vi "Sandbox HI Press.vi"() -> ()   [LabVIEW 2019]
uses:
  FPGA_API_class/FPGA API.lvclass
  FPGA/TypeDef/DO index.ctl
  <vilib>/Platform/TimedLoop/XDataNode/timing_clust.ctl
  <vilib>/Platform/TimedLoop/XDataNode/nitl_modes.ctl
  <vilib>/Platform/TimedLoop/XDataNode/wakeup.ctl
  Database_Postgress_class/Database_Postgress.lvclass
  D:/H4000/src/DatabaseInterface_class/DatabaseInterface.lvclass
  Database_Postgress_class/Connection Info.ctl
  Logger_class/Logger.lvclass
  ConfigJSON_class/ConfigJSON.lvclass
  D:/H4000/src/ConfigInterface_class/ConfigInterface.lvclass
  ConfigJSON_class/ConfigJSON.lvclass/ConfigJSON.ctl
  MessageAMC_class/MessageAMC.lvclass
  D:/H4000/src/MessageInterface_class/MessageInterface.lvclass
  Sig_AI_class/Sig_AI.lvclass
  D:/H4000/src/Proccess_class/Proccess.lvclass
  Sig_AI_class/Sig_AI.lvclass/Sig_AI.ctl
  Proccess_class/Proccess.lvclass/Proccess.ctl
  Logger_class/Logger.lvclass/Logger.ctl
  AnalogComparator_class/AnalogComparator.lvclass/AnalogComparator.ctl
  f5bc6a8b-969d-497a-8a5c-051cf4284504.vi
  ecb9b5e4-2695-48ff-9181-73dd1b10c553.vi
  af552bff-813f-42b3-9aac-38add1df6ad3.vi
  598a9a7a-3cbd-43cc-b63b-695f4522b225.vi
  Sig_AI_class/private/WriteToDb.vi
  Sig_AI_class/HandleRanges.vi
  Sig_AI_class/HandleAlarms.vi
  subvis/Scale_Raw_to_EU.vi
  AnalogComparator_class/GetStatus.vi
  AnalogComparator_class/GetTh.vi
  Logger_class/Enqueue Signal.vi
  Proccess_class/Read TagName.vi
  Proccess_class/Read Logger.vi
  AnalogComparator_class/SetValue.vi
  AnalogComparator_class/HandleDb.vi
  <vilib>/platform/TimedLoop/XDataNode/XDataNode.xnode
  <vilib>/Platform/TimedLoop/XDataNode/XDNodeRunTimeDep.lvlib
  Proccess_class/Proccess.lvclass
  DatabaseInterface_class/DatabaseInterface.lvclass
  <vilib>/ptbypt/NI_PtbyPt.lvlib
panel:
  in  "Time, ms":u32
  in  "Impulse open":bool
  out "x > y? 2":bool
  out "x > y?":bool
  out "Waveform Chart 4":dbl[][](graph)
  out "Waveform Chart 3":dbl(graph)
  out "Waveform Chart 2":dbl[][](graph)
  out "error out":errorcluster
  out "Iteration Duration":i64
  in  "Enable Stop Drive":bool
  in  "Enable Close Outlet":bool
  in  "Enable Close Inlet":bool
  out "SP RAW":dbl
  out "Waveform Chart":cluster{"SP":dbl, "Scaled":dbl}(graph)
  out "AI 6":dbl caption="Давление в образце\n[AI 6]"
  out "AI 5":dbl caption="Давление после насоса \nвысокого давления [AI 5]"
  out "AI 9":dbl caption="Давление  в  линии подачи \nвоздуха после БПВ [AI 9]"
  out "AI 8":dbl caption="Давление  в  линии подачи \nвоздуха в БПВ [AI 8]"
  out "AI4":dbl caption="ОС от клапана \n[AI 4]"
  out "DO 14":bool caption="Y29.10  \n33.6\nDO14"
  out "DO 17":bool caption="33.3\nY29.13\nDO17"
  out "DO 6":bool caption="33.8\nY29.2\nDO6"
  out "DO 9":bool caption="33.1\nY29.5\nDO9"
  out "19":bool caption="AIR"
  in  "SP 2":dbl
  in  "stop":bool
  in  "ALARM":bool
  in  "SP":dbl
  in  "GO DOWN":bool
  in  "GP UP":bool
  in  "AIR":bool
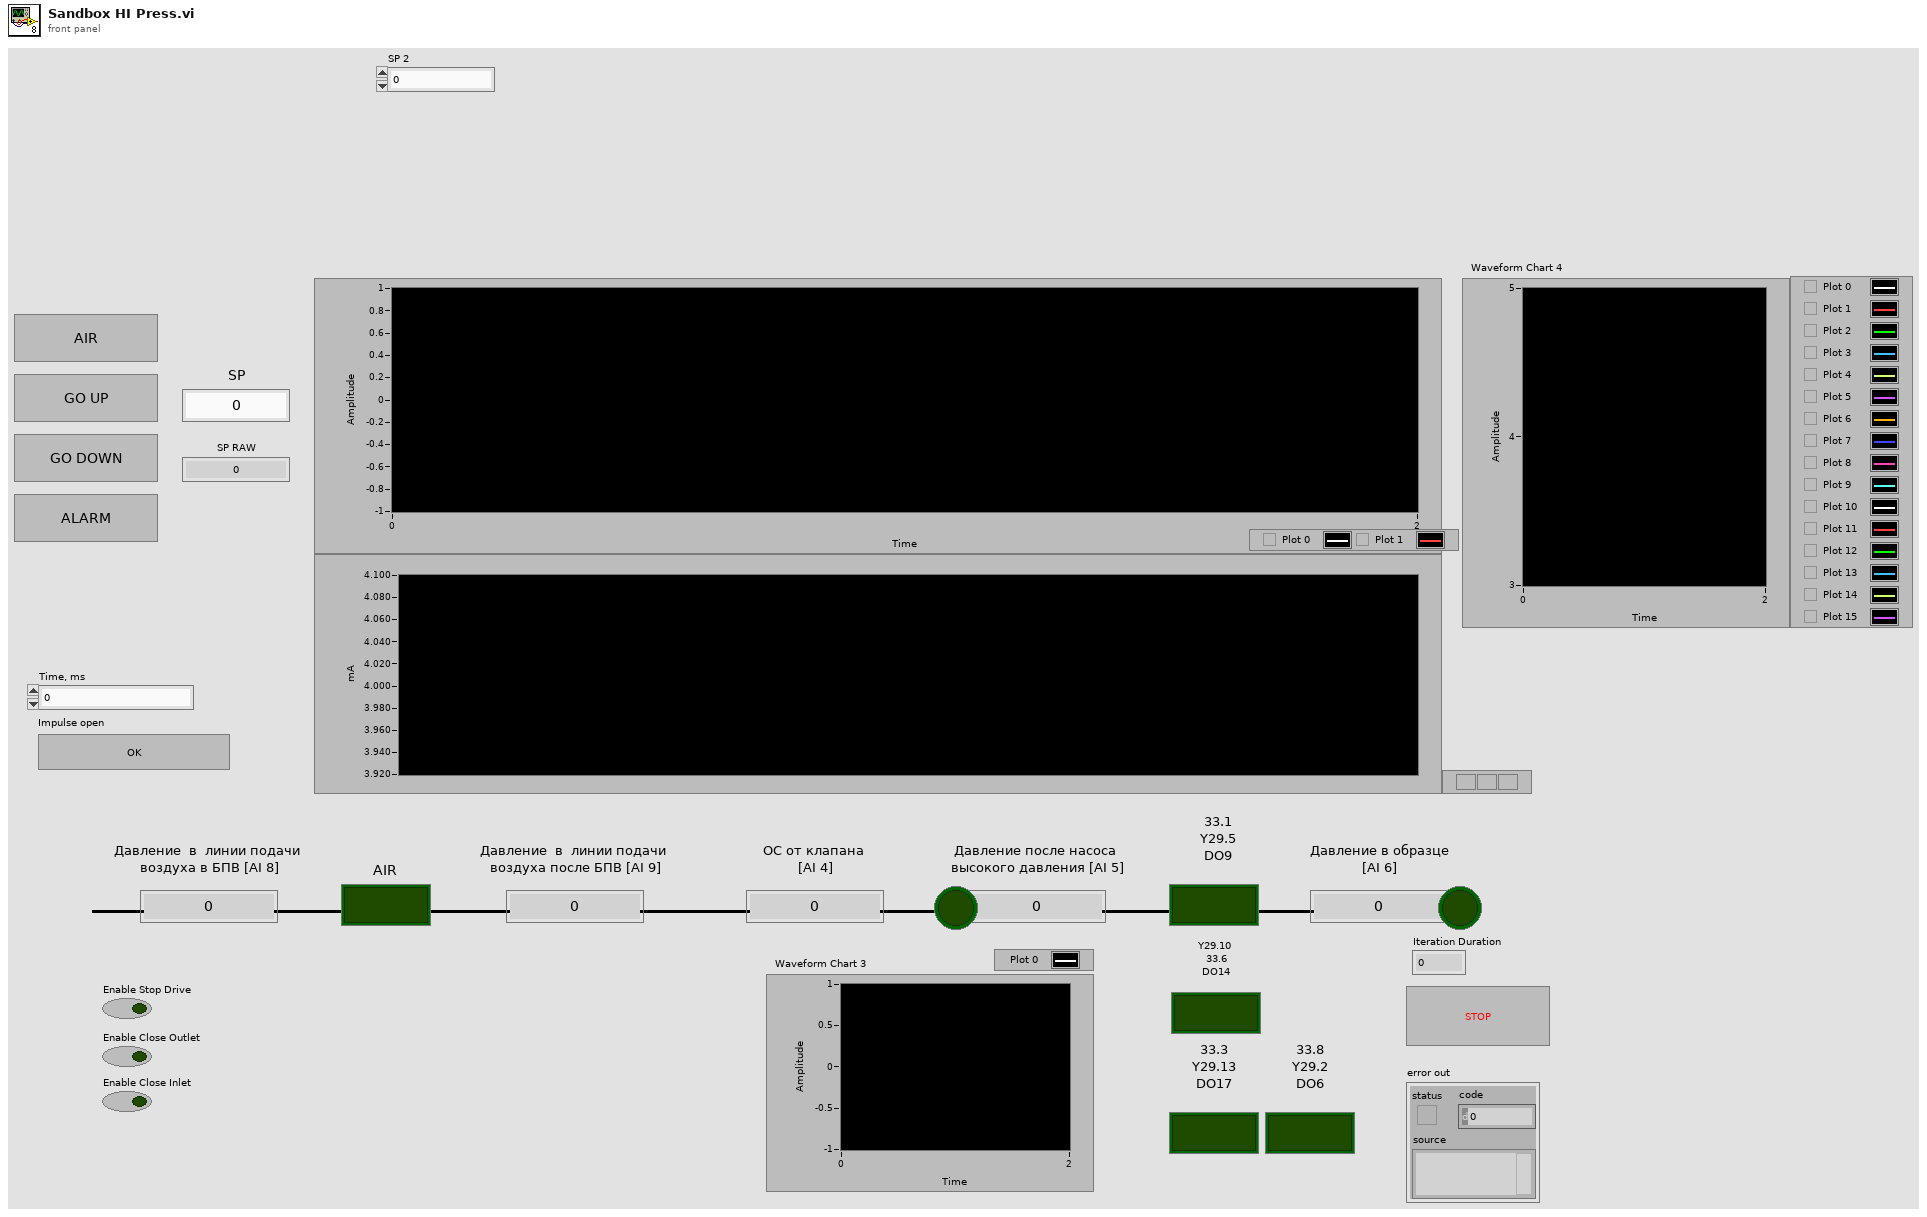
[diagram p1: front panel]
types:
  T1 = typedef "DO index.ctl" = u8
  T2 = typedef "DatabaseInterface.lvclass/Connection Info.ctl" = cluster{"IP_Address":string, "Port":u16, "Timeout":i32, "User":string, "Password":string, "Database":string}
  T3 = typedef "XDNodeRunTimeDep.lvlib/timing_clust.ctl" = cluster{"Expected End [f-1]":u64, "Actual End [f-1]":u64, "Finished Late? [f-1]":bool, "Expected End [i-1]":u64, "Actual End [i-1]":u64, "Finished Late? [i-1]":bool, "Expected Start [i]":u64, "Actual Start [i]":u64, "Expected Start [f]":u64, "Actual Start [f]":u64, "Source Name":string, "Structure Name":string, "Period":i64, "Deadline":i64, "Offset":i64, "Start":i64, "Priority":i32, "Timeout":i32, "Mode":T4, "Wakeup Reason":T5, "Error":errorcluster, "Source Type":string, "Secondary Source Type":string, "Global End Time":u64, "Global Start Time":u64, "Frame Duration":u64, "Iteration Duration":u64, "Assigned CPU":i32, "I/O Scan Engine Mode":u32}
  T4 = typedef "XDNodeRunTimeDep.lvlib/nitl_modes.ctl" = enum32{"No Change", "Process missed periods, maintain original phase", "Discard missed periods, maintain original phase", "Process missed periods, ignore original phase", "Discard missed periods, ignore original phase"}
  T5 = typedef "XDNodeRunTimeDep.lvlib/wakeup.ctl" = enum32{"Normal", "Aborted", "Asynchronous wakeup", "Timing source error", "Timed loop error", "Timeout"}
  T6 = typedef "AI_Data.ctl" = cluster{"Raw":dbl, "Scaled":dbl, "OutOfRangeMax":bool, "OutOfRangeMin":bool, "HIHI":bool, "HI":bool, "LO":bool, "LOLO":bool, "OutOfRangeMax_val":dbl, "OutOfRangeMin_val":dbl, "HIHI_val":dbl, "HI_val":dbl, "LO_val":dbl, "LOLO_val":dbl}
  T7 = typedef "Config_Scale.ctl" = cluster{"scale [EU/RAW]":dbl, "offset [EU]":dbl}
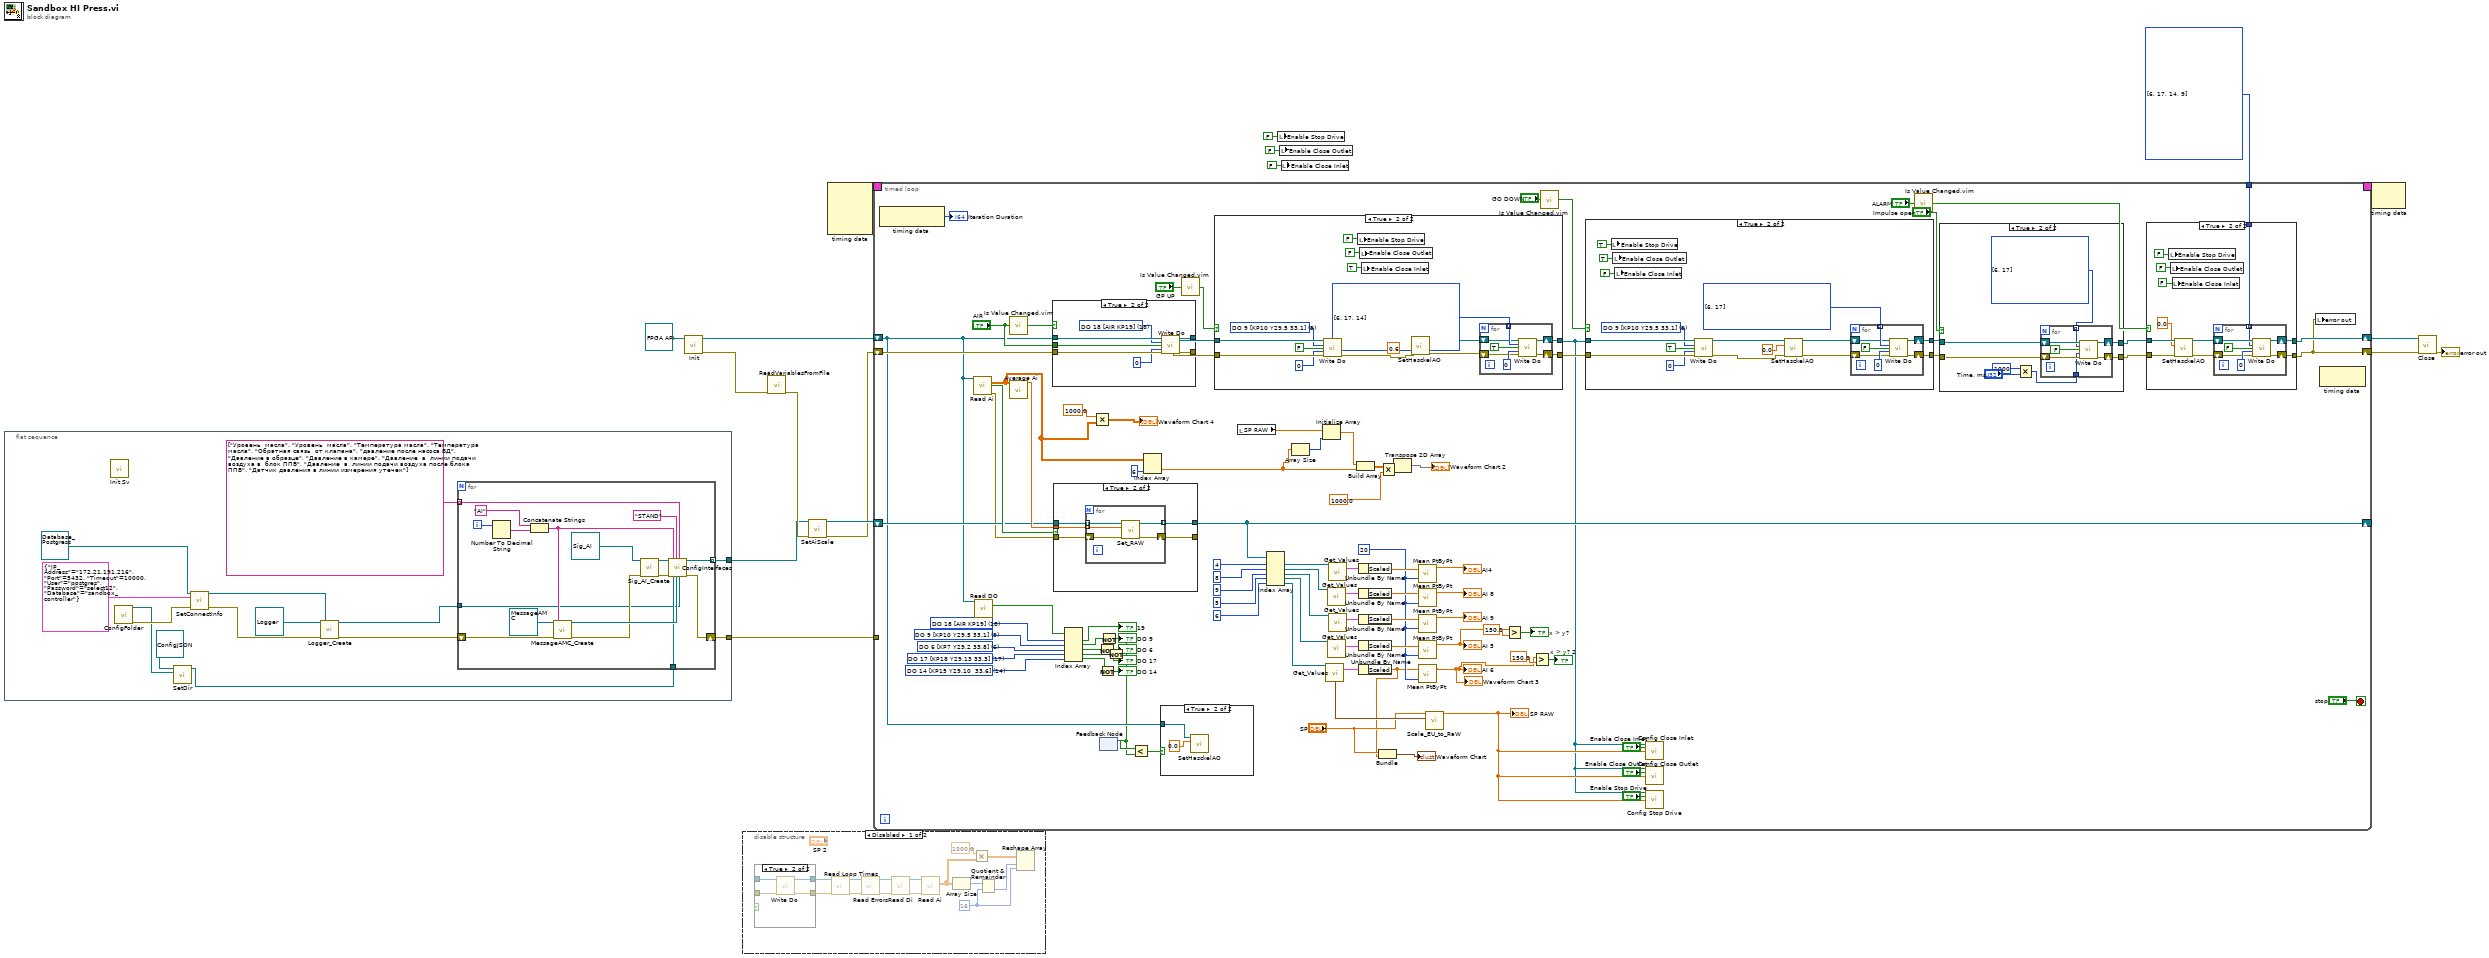
[diagram p0: block diagram]
diagram:
  w1 = T1[] [6, 17, 14, 9] items=["DO 0 [KP1 [DO 0]]", "DO 1 [ON KP2 [DO 1]]", "DO 2 [ON KP3 [DO 2]]", "DO 3 [WATER Y18.1 [DO3]]", "DO 4 [WATER Y18.2 [DO4]]", "DO 5 [KP6 Y29.1 33.7]", "DO 6 [KP7 Y29.2 33.8]", "DO 7 [KP8 Y29.3 33.9]", "DO 8 [KP9 Y29.4  33.12]", "DO 9 [KP10 Y29.5 33.1]", "DO 10 [KP11 Y29.6 33.2]", "DO 11 [KP12 Y29.7  33.13]", "DO 12 [KP13 Y29.8  33.11]", "DO 13 [KP14 Y29.9 33.10]", "DO 14 [KP15 Y29.10  33.6]", "DO 15 [KP16 Y29.11  33.5]", "DO 16 [KP17 Y29.12  33.4]", "DO 17 [KP18 Y29.13 33.3]", "DO 18 [AIR KP19]", "DO 19 [STEP DRIVE EN KP20]", "DO 20 [KP21 Y44.1 OPEN]", "DO 21 [ KP22 Y44.1 CLOSE]", "DO 22 [ KP23 Y44.2 OPEN]", "DO 23", "DO 24 [STEP DRIVE 1]", "DO 25 [STEP DRIVE 2]"] ("#DO")
  n1 = flat-sequence {
    tunnel: [w19] -> w8
    tunnel: [w18] -> w11
    frame #0 {
      n2 = call "Init Sv.vi"() -> ()  [unwired: 16 in]
      n3 = call "ConfigFolder.vi"() -> ("dup path"=w29:path, "error out"=w30:errorcluster)  [unwired: 14 in]
      n4 = call "SetDir.vi"("reference in"=refnum<class "ConfigJSON.lvclass"> refnum ("ConfigJSON"), "Config Dir"=w29) -> ("JSON"=w22:refnum<class "ConfigJSON.lvclass">)  [unwired: 13 in]
      n5 = call-dynamic "SetConnectInfo.vi"("reference in"=refnum<class "Database_Postgress.lvclass"> refnum, "Connection Info"=T2 {"IP_Address"="172.21.191.216", "Port"=5432, "Timeout"=10000, "User"="postgres", "Password"="select12", "Database"="sandbox_controller"}, "error in (no error)"=w30) -> ("reference out"=w27:refnum<class "Database_Postgress.lvclass">, "error out"=w28:errorcluster)  [unwired: 11 in]
      n6 = call "Logger_Create.vi"("reference in"=refnum<class "Logger.lvclass"> refnum, "error in (no error)"=w28, "DatabaseInterface"=w27) -> ("reference out"=w21:refnum<class "Logger.lvclass">, "error out"=w20:errorcluster)  [unwired: 15 in]
      n7 = for {
        tunnel: [w42] -> w19 mode=indexing
        shift-right: [w43] -> w18
        shift-left: w20 -> [w45]
        tunnel: string[] ["Уровень  масла", "Уровень  масла", "Температура масла", "Температура масла", "Обратная связь  от клапана", "давление после насоса ВД", "Давление в образце", "Давление в камере", "Давление  в  линии подачи воздуха в  блок ППВ", "Давление  в  линии подачи воздуха после блока ППВ", "Датчик давления в линии измерения утечек"] ("ParentName") -> [w34] mode=indexing
        tunnel: w22 -> [w33]
        tunnel: w21 -> [w32]
        i -> [w48]
        n8 = Number To Decimal String(number=w48) -> (decimal integer string=w47:string)  [unwired: 1 in]
        n9 = Concatenate Strings("AI" ("string"), w47) -> (w35:string)
        n10 = call "MessageAMC_Create.vi"("reference in"=refnum<class "MessageAMC.lvclass"> refnum, "error in (no error)"=w45, "message queue name"=w35) -> ("amc"=w40:refnum<class "MessageAMC.lvclass">, "error out"=w36:errorcluster)  [unwired: 15 in]
        n11 = call "Sig_AI_Create.vi"("reference in"=refnum<class "Sig_AI.lvclass"> refnum ("Sig_AI"), "error in (no error)"=w36) -> ("reference out"=w38:refnum<class "Sig_AI.lvclass">, "error out"=w37:errorcluster)  [unwired: 16 in]
        n12 = call "ConfigInterfaces.vi"("reference in"=w38, "error in (no error)"=w37, "Name"=w35, "ConfigInterface"=w33, "ParentName"="STAND", "MessageInterface"=w40, "Description"=w34, "Logger"=w32) -> ("reference out"=w42:refnum<class "Sig_AI.lvclass">, "error out"=w43:errorcluster)  [unwired: 10 in]
      }
    }
  }
  n13 = call "Init.vi"("FPGA API in"=refnum<class "FPGA API.lvclass"> refnum) -> ("FPGA API out"=w16:refnum<class "FPGA API.lvclass">, "error out"=w10:errorcluster)  [unwired: 13 in]
  n14 = disable-structure shown="Disabled" {
    frame Disabled {
      w49 = 16 ("dimension size")
      n15 = case shown="True" {
        selector: _ -> [_ _]
        tunnel: [w64 w68] -> w51
        tunnel: [w63 w67] -> w52
        tunnel: _ -> [w64 w65]
        tunnel: _ -> [w63 w66]
        frame False {
        }
        frame True {
          n16 = call "Write Do.vi"("FPGA API in"=w65, "error in (no error)"=w66) -> ("FPGA API out"=w68:refnum<class "FPGA API.lvclass">, "error out"=w67:errorcluster)  [unwired: 12 in]
        }
      }
      n17 = call "Read Loop Times.vi"("FPGA API in"=w51, "error in (no error)"=w52) -> ("FPGA API out"=w54:refnum<class "FPGA API.lvclass">, "error out"=w53:errorcluster)  [unwired: 9 in, 3 out]
      n18 = call "Read Errors.vi"("FPGA API in"=w54, "error in (no error)"=w53) -> ("FPGA API out"=w55:refnum<class "FPGA API.lvclass">, "error out"=w56:errorcluster)  [unwired: 8 in, 4 out]
      n19 = call "Read Di.vi"("FPGA API in"=w55, "error in (no error)"=w56) -> ("FPGA API out"=w58:refnum<class "FPGA API.lvclass">, "error out"=w57:errorcluster)  [unwired: 11 in, 1 out]
      n20 = call "Read Ai.vi"("FPGA API in"=w58, "error in (no error)"=w57) -> ("AI Data"=w59:dbl[][])  [unwired: 10 in, 3 out]
      n21 = Array Size(array=w59) -> (size(s)=w60:i32[])
      n22 = Multiply(x=1000.0, y=w59) -> (x*y=w61:dbl[][])
      n23 = Quotient & Remainder(x=w60, y=w49) -> (floor(x/y)=w62:i32[])  [unwired: 1 out]
      n24 = Reshape Array(w61, w62, w49) -> ()  [unwired: 1 out]
    }
    frame Enabled {
    }
  }
  n25 = call "ReadVariablesFromFile.vi"("error in (no error)"=w10) -> ("error out"=w9:errorcluster)  [unwired: 14 in]
  n26 = call "SetAiScale.vi"("Array"=w8, "error in (no error)"=w9) -> ("Array 2"=w7:refnum<class "Sig_AI.lvclass">[], "error out"=w6:errorcluster)  [unwired: 12 in]
  n27 = node-c288() -> (w13:T3)  [unwired: 4 in]
  n28 = timed-loop {
    shift-right: [w111] -> w15
    shift-left: w16 -> [w103]
    shift-right: [w99] -> w14
    shift-left: w6 -> [w162]
    timing: w13 -> [_]
    timing-out: [_] -> w12
    tunnel: w11 -> [_]
    shift-right: [w138] -> _
    shift-left: w7 -> [w155]
    tunnel: w1 -> [w112]
    stop <- "stop" stop-if-true
    w115 = 20 ("sample length")
    w139 = T1 14 items=["DO 0 [KP1 [DO 0]]", "DO 1 [ON KP2 [DO 1]]", "DO 2 [ON KP3 [DO 2]]", "DO 3 [WATER Y18.1 [DO3]]", "DO 4 [WATER Y18.2 [DO4]]", "DO 5 [KP6 Y29.1 33.7]", "DO 6 [KP7 Y29.2 33.8]", "DO 7 [KP8 Y29.3 33.9]", "DO 8 [KP9 Y29.4  33.12]", "DO 9 [KP10 Y29.5 33.1]", "DO 10 [KP11 Y29.6 33.2]", "DO 11 [KP12 Y29.7  33.13]", "DO 12 [KP13 Y29.8  33.11]", "DO 13 [KP14 Y29.9 33.10]", "DO 14 [KP15 Y29.10  33.6]", "DO 15 [KP16 Y29.11  33.5]", "DO 16 [KP17 Y29.12  33.4]", "DO 17 [KP18 Y29.13 33.3]", "DO 18 [AIR KP19]", "DO 19 [STEP DRIVE EN KP20]", "DO 20 [KP21 Y44.1 OPEN]", "DO 21 [ KP22 Y44.1 CLOSE]", "DO 22 [ KP23 Y44.2 OPEN]", "DO 23", "DO 24 [STEP DRIVE 1]", "DO 25 [STEP DRIVE 2]"] ("#DO")
    w146 = T1 17 items=["DO 0 [KP1 [DO 0]]", "DO 1 [ON KP2 [DO 1]]", "DO 2 [ON KP3 [DO 2]]", "DO 3 [WATER Y18.1 [DO3]]", "DO 4 [WATER Y18.2 [DO4]]", "DO 5 [KP6 Y29.1 33.7]", "DO 6 [KP7 Y29.2 33.8]", "DO 7 [KP8 Y29.3 33.9]", "DO 8 [KP9 Y29.4  33.12]", "DO 9 [KP10 Y29.5 33.1]", "DO 10 [KP11 Y29.6 33.2]", "DO 11 [KP12 Y29.7  33.13]", "DO 12 [KP13 Y29.8  33.11]", "DO 13 [KP14 Y29.9 33.10]", "DO 14 [KP15 Y29.10  33.6]", "DO 15 [KP16 Y29.11  33.5]", "DO 16 [KP17 Y29.12  33.4]", "DO 17 [KP18 Y29.13 33.3]", "DO 18 [AIR KP19]", "DO 19 [STEP DRIVE EN KP20]", "DO 20 [KP21 Y44.1 OPEN]", "DO 21 [ KP22 Y44.1 CLOSE]", "DO 22 [ KP23 Y44.2 OPEN]", "DO 23", "DO 24 [STEP DRIVE 1]", "DO 25 [STEP DRIVE 2]"] ("#DO")
    w147 = T1 6 items=["DO 0 [KP1 [DO 0]]", "DO 1 [ON KP2 [DO 1]]", "DO 2 [ON KP3 [DO 2]]", "DO 3 [WATER Y18.1 [DO3]]", "DO 4 [WATER Y18.2 [DO4]]", "DO 5 [KP6 Y29.1 33.7]", "DO 6 [KP7 Y29.2 33.8]", "DO 7 [KP8 Y29.3 33.9]", "DO 8 [KP9 Y29.4  33.12]", "DO 9 [KP10 Y29.5 33.1]", "DO 10 [KP11 Y29.6 33.2]", "DO 11 [KP12 Y29.7  33.13]", "DO 12 [KP13 Y29.8  33.11]", "DO 13 [KP14 Y29.9 33.10]", "DO 14 [KP15 Y29.10  33.6]", "DO 15 [KP16 Y29.11  33.5]", "DO 16 [KP17 Y29.12  33.4]", "DO 17 [KP18 Y29.13 33.3]", "DO 18 [AIR KP19]", "DO 19 [STEP DRIVE EN KP20]", "DO 20 [KP21 Y44.1 OPEN]", "DO 21 [ KP22 Y44.1 CLOSE]", "DO 22 [ KP23 Y44.2 OPEN]", "DO 23", "DO 24 [STEP DRIVE 1]", "DO 25 [STEP DRIVE 2]"] ("#DO")
    w148 = T1 9 items=["DO 0 [KP1 [DO 0]]", "DO 1 [ON KP2 [DO 1]]", "DO 2 [ON KP3 [DO 2]]", "DO 3 [WATER Y18.1 [DO3]]", "DO 4 [WATER Y18.2 [DO4]]", "DO 5 [KP6 Y29.1 33.7]", "DO 6 [KP7 Y29.2 33.8]", "DO 7 [KP8 Y29.3 33.9]", "DO 8 [KP9 Y29.4  33.12]", "DO 9 [KP10 Y29.5 33.1]", "DO 10 [KP11 Y29.6 33.2]", "DO 11 [KP12 Y29.7  33.13]", "DO 12 [KP13 Y29.8  33.11]", "DO 13 [KP14 Y29.9 33.10]", "DO 14 [KP15 Y29.10  33.6]", "DO 15 [KP16 Y29.11  33.5]", "DO 16 [KP17 Y29.12  33.4]", "DO 17 [KP18 Y29.13 33.3]", "DO 18 [AIR KP19]", "DO 19 [STEP DRIVE EN KP20]", "DO 20 [KP21 Y44.1 OPEN]", "DO 21 [ KP22 Y44.1 CLOSE]", "DO 22 [ KP23 Y44.2 OPEN]", "DO 23", "DO 24 [STEP DRIVE 1]", "DO 25 [STEP DRIVE 2]"] ("#DO")
    w152 = T1 18 items=["DO 0 [KP1 [DO 0]]", "DO 1 [ON KP2 [DO 1]]", "DO 2 [ON KP3 [DO 2]]", "DO 3 [WATER Y18.1 [DO3]]", "DO 4 [WATER Y18.2 [DO4]]", "DO 5 [KP6 Y29.1 33.7]", "DO 6 [KP7 Y29.2 33.8]", "DO 7 [KP8 Y29.3 33.9]", "DO 8 [KP9 Y29.4  33.12]", "DO 9 [KP10 Y29.5 33.1]", "DO 10 [KP11 Y29.6 33.2]", "DO 11 [KP12 Y29.7  33.13]", "DO 12 [KP13 Y29.8  33.11]", "DO 13 [KP14 Y29.9 33.10]", "DO 14 [KP15 Y29.10  33.6]", "DO 15 [KP16 Y29.11  33.5]", "DO 16 [KP17 Y29.12  33.4]", "DO 17 [KP18 Y29.13 33.3]", "DO 18 [AIR KP19]", "DO 19 [STEP DRIVE EN KP20]", "DO 20 [KP21 Y44.1 OPEN]", "DO 21 [ KP22 Y44.1 CLOSE]", "DO 22 [ KP23 Y44.2 OPEN]", "DO 23", "DO 24 [STEP DRIVE 1]", "DO 25 [STEP DRIVE 2]"] ("#DO")
    n29 = node-c288() -> (→"Iteration Duration":i64)  [unwired: 1 in]
    n30 = call "Read Ai.vi"("FPGA API in"=w103) -> ("AI Data"=w82:dbl[][], "Valud Data"=w157:bool, "error out"=w154:errorcluster)  [unwired: 11 in, 1 out]
    n31 = call "Read DO.vi"("FPGA API in"=w103) -> ("Ds"=w153:bool[])  [unwired: 12 in, 2 out]
    n32 = call "Average Ai.vi"("AIs"=w82) -> ("Array"=w156:dbl[])  [unwired: 14 in]
    n33 = call "Is Value Changed.vim"("value"="AIR") -> ("changed or first call?"=w160:bool)
    n34 = case shown="True" w160 {
      tunnel: [w269 w276] -> w159
      tunnel: [w268 w275] -> w158
      tunnel: w103 -> [w269 w273]
      tunnel: w162 -> [w268 w274]
      tunnel: "AIR" -> [_ w272]
      frame False {
      }
      frame True {
        w271 = T1 18 items=["DO 0 [KP1 [DO 0]]", "DO 1 [ON KP2 [DO 1]]", "DO 2 [ON KP3 [DO 2]]", "DO 3 [WATER Y18.1 [DO3]]", "DO 4 [WATER Y18.2 [DO4]]", "DO 5 [KP6 Y29.1 33.7]", "DO 6 [KP7 Y29.2 33.8]", "DO 7 [KP8 Y29.3 33.9]", "DO 8 [KP9 Y29.4  33.12]", "DO 9 [KP10 Y29.5 33.1]", "DO 10 [KP11 Y29.6 33.2]", "DO 11 [KP12 Y29.7  33.13]", "DO 12 [KP13 Y29.8  33.11]", "DO 13 [KP14 Y29.9 33.10]", "DO 14 [KP15 Y29.10  33.6]", "DO 15 [KP16 Y29.11  33.5]", "DO 16 [KP17 Y29.12  33.4]", "DO 17 [KP18 Y29.13 33.3]", "DO 18 [AIR KP19]", "DO 19 [STEP DRIVE EN KP20]", "DO 20 [KP21 Y44.1 OPEN]", "DO 21 [ KP22 Y44.1 CLOSE]", "DO 22 [ KP23 Y44.2 OPEN]", "DO 23", "DO 24 [STEP DRIVE 1]", "DO 25 [STEP DRIVE 2]"] ("#DO")
        n35 = call "Write Do.vi"("FPGA API in"=w273, "#DO"=w271, "value"=w272, "Time uSec"=u32 0, "error in (no error)"=w274) -> ("FPGA API out"=w276:refnum<class "FPGA API.lvclass">, "error out"=w275:errorcluster)  [unwired: 9 in]
      }
    }
    n36 = case shown="True" w157 {
      tunnel: [w256 w262] -> _
      tunnel: [w257 w261] -> w138
      tunnel: w156 -> [_ w260]
      tunnel: w155 -> [w257 w259]
      tunnel: w154 -> [w256 w258]
      frame False {
      }
      frame True {
        n37 = for {
          shift-right: [w266] -> w262
          shift-left: w258 -> [w267]
          tunnel: [w265] -> w261 mode=indexing
          tunnel: w260 -> [w264] mode=indexing
          tunnel: w259 -> [w263] mode=indexing
          n38 = call "Set_RAW.vi"("reference in"=w263, "RAW"=w264, "error in (no error)"=w267) -> ("reference out"=w265:refnum<class "Sig_AI.lvclass">, "error out"=w266:errorcluster)  [unwired: 11 in]
        }
      }
    }
    n39 = Index Array(array=w153, index #1=w152, index #2=w148, index #3=w147, index #4=w146, index #5=w139) -> (element #1=→"19":bool, element #2=w101:bool, element #3=w145:bool, element #4=w144:bool, element #5=w140:bool)
    n40 = Multiply(x=1000.0, y=w82) -> (x*y=→"Waveform Chart 4":dbl[][])
    n41 = Not(x=w145) -> (.not. x?=→"DO 6":bool)
    n42 = Not(x=w140) -> (.not. x?=→"DO 14":bool)
    n43 = feedback #1() -> (w102:bool)  [unwired: 1 in]
    n44 = Not(x=w101) -> (.not. x?=w95:bool)
    "DO 9" <- w95
    n45 = feedback-in #1(w95) -> ()
    n46 = Not(x=w144) -> (.not. x?=→"DO 17":bool)
    n47 = Less?(x=w102, y=w95) -> (x < y?=w100:bool)
    n48 = Index Array(array=w82, index (col)=6 ("disabled index (col)")) -> (element=w89:dbl[])  [unwired: 1 in]
    n49 = case shown="True" w100 {
      tunnel: w103 -> [_ w181]
      frame False {
      }
      frame True {
        n50 = call "SetHasckelAO.vi"("FPGA API in"=w181, "Haskel in"=0.0) -> ()  [unwired: 12 in, 2 out]
      }
    }
    n51 = call "Is Value Changed.vim"("value"="GP UP") -> ("changed or first call?"=w150:bool)
    n52 = case shown="True" w150 {
      tunnel: [w184 w194] -> w108
      tunnel: [w183 w193] -> w142
      tunnel: w159 -> [w184 w199]
      tunnel: w158 -> [w183 w200]
      frame False {
      }
      frame True {
        w195 = T1[] [6, 17, 14] items=["DO 0 [KP1 [DO 0]]", "DO 1 [ON KP2 [DO 1]]", "DO 2 [ON KP3 [DO 2]]", "DO 3 [WATER Y18.1 [DO3]]", "DO 4 [WATER Y18.2 [DO4]]", "DO 5 [KP6 Y29.1 33.7]", "DO 6 [KP7 Y29.2 33.8]", "DO 7 [KP8 Y29.3 33.9]", "DO 8 [KP9 Y29.4  33.12]", "DO 9 [KP10 Y29.5 33.1]", "DO 10 [KP11 Y29.6 33.2]", "DO 11 [KP12 Y29.7  33.13]", "DO 12 [KP13 Y29.8  33.11]", "DO 13 [KP14 Y29.9 33.10]", "DO 14 [KP15 Y29.10  33.6]", "DO 15 [KP16 Y29.11  33.5]", "DO 16 [KP17 Y29.12  33.4]", "DO 17 [KP18 Y29.13 33.3]", "DO 18 [AIR KP19]", "DO 19 [STEP DRIVE EN KP20]", "DO 20 [KP21 Y44.1 OPEN]", "DO 21 [ KP22 Y44.1 CLOSE]", "DO 22 [ KP23 Y44.2 OPEN]", "DO 23", "DO 24 [STEP DRIVE 1]", "DO 25 [STEP DRIVE 2]"] ("#DO")
        w198 = T1 9 items=["DO 0 [KP1 [DO 0]]", "DO 1 [ON KP2 [DO 1]]", "DO 2 [ON KP3 [DO 2]]", "DO 3 [WATER Y18.1 [DO3]]", "DO 4 [WATER Y18.2 [DO4]]", "DO 5 [KP6 Y29.1 33.7]", "DO 6 [KP7 Y29.2 33.8]", "DO 7 [KP8 Y29.3 33.9]", "DO 8 [KP9 Y29.4  33.12]", "DO 9 [KP10 Y29.5 33.1]", "DO 10 [KP11 Y29.6 33.2]", "DO 11 [KP12 Y29.7  33.13]", "DO 12 [KP13 Y29.8  33.11]", "DO 13 [KP14 Y29.9 33.10]", "DO 14 [KP15 Y29.10  33.6]", "DO 15 [KP16 Y29.11  33.5]", "DO 16 [KP17 Y29.12  33.4]", "DO 17 [KP18 Y29.13 33.3]", "DO 18 [AIR KP19]", "DO 19 [STEP DRIVE EN KP20]", "DO 20 [KP21 Y44.1 OPEN]", "DO 21 [ KP22 Y44.1 CLOSE]", "DO 22 [ KP23 Y44.2 OPEN]", "DO 23", "DO 24 [STEP DRIVE 1]", "DO 25 [STEP DRIVE 2]"] ("#DO")
        n53 = call "Write Do.vi"("FPGA API in"=w199, "#DO"=w198, "value"=FALSE, "Time uSec"=u32 0, "error in (no error)"=w200) -> ("FPGA API out"=w191:refnum<class "FPGA API.lvclass">, "error out"=w190:errorcluster)  [unwired: 9 in]
        n54 = local write "Enable Stop Drive"(FALSE ("Enable Stop Drive")) -> ()
        n55 = local write "Enable Close Outlet"(FALSE ("Enable Close Outlet")) -> ()
        n56 = local write "Enable Close Inlet"(TRUE ("Enable Close Inlet")) -> ()
        n57 = call "SetHasckelAO.vi"("FPGA API in"=w191, "Haskel in"=0.6, "error in (no error)"=w190) -> ("FPGA API out"=w188:refnum<class "FPGA API.lvclass">, "error out"=w189:errorcluster)  [unwired: 11 in]
        n58 = for {
          tunnel: w195 -> [w205] mode=indexing
          shift-right: [w202] -> w194
          shift-left: w188 -> [w204]
          shift-right: [w201] -> w193
          shift-left: w189 -> [w203]
          n59 = call "Write Do.vi"("FPGA API in"=w204, "#DO"=w205, "value"=TRUE, "Time uSec"=u32 0, "error in (no error)"=w203) -> ("FPGA API out"=w202:refnum<class "FPGA API.lvclass">, "error out"=w201:errorcluster)  [unwired: 9 in]
        }
      }
    }
    n60 = local read "SP RAW"() -> (w90:dbl)
    n61 = Index Array(array=w138, index #1=4 ("index"), index #2=8 ("index"), index #3=9 ("index"), index #4=5 ("index"), index #5=6 ("index")) -> (element #1=w132:refnum<class "Sig_AI.lvclass">, element #2=w126:refnum<class "Sig_AI.lvclass">, element #3=w125:refnum<class "Sig_AI.lvclass">, element #4=w124:refnum<class "Sig_AI.lvclass">, element #5=w123:refnum<class "Sig_AI.lvclass">)
    n62 = Array Size(array=w89) -> (size(s)=w88:i32)
    n63 = Initialize Array(w90, w88) -> (w87:dbl[])
    n64 = call "Get_Values.vi"("reference in"=w123) -> ("Data"=w127:T6, "Scale"=w110:T7)  [unwired: 13 in]
    n65 = call "Get_Values.vi"("reference in"=w124) -> ("Data"=w128:T6)  [unwired: 13 in, 1 out]
    n66 = call "Get_Values.vi"("reference in"=w126) -> ("Data"=w130:T6)  [unwired: 13 in, 1 out]
    n67 = call "Get_Values.vi"("reference in"=w132) -> ("Data"=w131:T6)  [unwired: 13 in, 1 out]
    n68 = call "Get_Values.vi"("reference in"=w125) -> ("Data"=w129:T6)  [unwired: 13 in, 1 out]
    n69 = Build Array(w87, w89) -> (w86:dbl[][])
    n70 = Unbundle By Name(w131) -> ("Scaled"=w122:dbl)
    n71 = Unbundle By Name(w130) -> ("Scaled"=w118:dbl)
    n72 = Unbundle By Name(w129) -> ("Scaled"=w119:dbl)
    n73 = Unbundle By Name(w128) -> ("Scaled"=w120:dbl)
    n74 = Unbundle By Name(w127) -> ("Scaled"=w93:dbl)
    n75 = Bundle("SP"="SP", "Scaled"=w93) -> (→"Waveform Chart":cluster{"SP":dbl, "Scaled":dbl})  [unwired: 1 in]
    n76 = Multiply(x=w86, y=1000.0) -> (x*y=w84:dbl[][])
    n77 = Transpose 2D Array(2D array=w84) -> (transposed array=→"Waveform Chart 2":dbl[][])
    n78 = call <vilib>:"Mean PtByPt.vi"("x"=w122, "sample length"=w115) -> ("mean"=→"AI4":dbl)  [unwired: 2 in, 1 out]
    n79 = call <vilib>:"Mean PtByPt.vi"("x"=w118, "sample length"=w115) -> ("mean"=→"AI 8":dbl)  [unwired: 2 in, 1 out]
    n80 = call <vilib>:"Mean PtByPt.vi"("x"=w119, "sample length"=w115) -> ("mean"=→"AI 9":dbl)  [unwired: 2 in, 1 out]
    n81 = call <vilib>:"Mean PtByPt.vi"("x"=w120, "sample length"=w115) -> ("mean"=w79:dbl)  [unwired: 2 in, 1 out]
    "AI 5" <- w79
    n82 = call <vilib>:"Mean PtByPt.vi"("x"=w93, "sample length"=w115) -> ("mean"=w75:dbl)  [unwired: 2 in, 1 out]
    "AI 6" <- w75
    "Waveform Chart 3" <- w75
    n83 = call "Scale_EU_to_RaW.vi"("ConfigScale"=w110, "EU"="SP") -> ("RAW"=w109:dbl)  [unwired: 9 in]
    "SP RAW" <- w109
    n84 = Greater?(x=w79, y=150.0 ("x")) -> (0:→"x > y?":bool)
    n85 = Greater?(x=w75, y=150.0 ("x")) -> (0:→"x > y? 2":bool)
    n86 = call "Is Value Changed.vim"("value"="GO DOWN") -> ("changed or first call?"=w143:bool)
    n87 = case shown="True" w143 {
      tunnel: [w232 w242] -> w73
      tunnel: [w231 w241] -> w72
      tunnel: w108 -> [w232 w247]
      tunnel: w142 -> [w231 w248]
      frame False {
      }
      frame True {
        w243 = T1[] [6, 17] items=["DO 0 [KP1 [DO 0]]", "DO 1 [ON KP2 [DO 1]]", "DO 2 [ON KP3 [DO 2]]", "DO 3 [WATER Y18.1 [DO3]]", "DO 4 [WATER Y18.2 [DO4]]", "DO 5 [KP6 Y29.1 33.7]", "DO 6 [KP7 Y29.2 33.8]", "DO 7 [KP8 Y29.3 33.9]", "DO 8 [KP9 Y29.4  33.12]", "DO 9 [KP10 Y29.5 33.1]", "DO 10 [KP11 Y29.6 33.2]", "DO 11 [KP12 Y29.7  33.13]", "DO 12 [KP13 Y29.8  33.11]", "DO 13 [KP14 Y29.9 33.10]", "DO 14 [KP15 Y29.10  33.6]", "DO 15 [KP16 Y29.11  33.5]", "DO 16 [KP17 Y29.12  33.4]", "DO 17 [KP18 Y29.13 33.3]", "DO 18 [AIR KP19]", "DO 19 [STEP DRIVE EN KP20]", "DO 20 [KP21 Y44.1 OPEN]", "DO 21 [ KP22 Y44.1 CLOSE]", "DO 22 [ KP23 Y44.2 OPEN]", "DO 23", "DO 24 [STEP DRIVE 1]", "DO 25 [STEP DRIVE 2]"] ("#DO")
        w246 = T1 9 items=["DO 0 [KP1 [DO 0]]", "DO 1 [ON KP2 [DO 1]]", "DO 2 [ON KP3 [DO 2]]", "DO 3 [WATER Y18.1 [DO3]]", "DO 4 [WATER Y18.2 [DO4]]", "DO 5 [KP6 Y29.1 33.7]", "DO 6 [KP7 Y29.2 33.8]", "DO 7 [KP8 Y29.3 33.9]", "DO 8 [KP9 Y29.4  33.12]", "DO 9 [KP10 Y29.5 33.1]", "DO 10 [KP11 Y29.6 33.2]", "DO 11 [KP12 Y29.7  33.13]", "DO 12 [KP13 Y29.8  33.11]", "DO 13 [KP14 Y29.9 33.10]", "DO 14 [KP15 Y29.10  33.6]", "DO 15 [KP16 Y29.11  33.5]", "DO 16 [KP17 Y29.12  33.4]", "DO 17 [KP18 Y29.13 33.3]", "DO 18 [AIR KP19]", "DO 19 [STEP DRIVE EN KP20]", "DO 20 [KP21 Y44.1 OPEN]", "DO 21 [ KP22 Y44.1 CLOSE]", "DO 22 [ KP23 Y44.2 OPEN]", "DO 23", "DO 24 [STEP DRIVE 1]", "DO 25 [STEP DRIVE 2]"] ("#DO")
        n88 = local write "Enable Stop Drive"(TRUE ("Enable Stop Drive")) -> ()
        n89 = local write "Enable Close Outlet"(TRUE ("Enable Close Outlet")) -> ()
        n90 = local write "Enable Close Inlet"(FALSE ("Enable Close Inlet")) -> ()
        n91 = call "Write Do.vi"("FPGA API in"=w247, "#DO"=w246, "value"=TRUE, "Time uSec"=u32 0, "error in (no error)"=w248) -> ("FPGA API out"=w239:refnum<class "FPGA API.lvclass">, "error out"=w236:errorcluster)  [unwired: 9 in]
        n92 = call "SetHasckelAO.vi"("FPGA API in"=w239, "Haskel in"=0.0, "error in (no error)"=w236) -> ("FPGA API out"=w238:refnum<class "FPGA API.lvclass">, "error out"=w237:errorcluster)  [unwired: 11 in]
        n93 = for {
          tunnel: w243 -> [w253] mode=indexing
          shift-right: [w250] -> w242
          shift-left: w238 -> [w252]
          shift-right: [w249] -> w241
          shift-left: w237 -> [w251]
          n94 = call "Write Do.vi"("FPGA API in"=w252, "#DO"=w253, "value"=FALSE, "Time uSec"=u32 0, "error in (no error)"=w251) -> ("FPGA API out"=w250:refnum<class "FPGA API.lvclass">, "error out"=w249:errorcluster)  [unwired: 9 in]
        }
      }
    }
    n95 = call "Config Close Inlet.vi"("FPGA API in"=w108, "Enable Close Inlet"="Enable Close Inlet", "SP Close Inlet"=w109) -> ()  [unwired: 11 in, 2 out]
    n96 = call "Config Close Outlet.vi"("FPGA API in"=w108, "Enable Close Outlet"="Enable Close Outlet", "SP Close Outlet"=w109) -> ()  [unwired: 11 in, 2 out]
    n97 = call "Config Stop Drive.vi"("FPGA API in"=w108, "Enable Stop Drive"="Enable Stop Drive", "SP Stop Drive"=w109) -> ()  [unwired: 11 in, 2 out]
    n98 = call "Is Value Changed.vim"("value"="ALARM") -> ("changed or first call?"=w114:bool)
    n99 = case shown="True" "Impulse open" {
      tunnel: [w165 w173] -> w71
      tunnel: [w164 w172] -> w70
      tunnel: w73 -> [w165 w171]
      tunnel: w72 -> [w164 w170]
      frame False {
      }
      frame True {
        w169 = T1[] [6, 17] items=["DO 0 [KP1 [DO 0]]", "DO 1 [ON KP2 [DO 1]]", "DO 2 [ON KP3 [DO 2]]", "DO 3 [WATER Y18.1 [DO3]]", "DO 4 [WATER Y18.2 [DO4]]", "DO 5 [KP6 Y29.1 33.7]", "DO 6 [KP7 Y29.2 33.8]", "DO 7 [KP8 Y29.3 33.9]", "DO 8 [KP9 Y29.4  33.12]", "DO 9 [KP10 Y29.5 33.1]", "DO 10 [KP11 Y29.6 33.2]", "DO 11 [KP12 Y29.7  33.13]", "DO 12 [KP13 Y29.8  33.11]", "DO 13 [KP14 Y29.9 33.10]", "DO 14 [KP15 Y29.10  33.6]", "DO 15 [KP16 Y29.11  33.5]", "DO 16 [KP17 Y29.12  33.4]", "DO 17 [KP18 Y29.13 33.3]", "DO 18 [AIR KP19]", "DO 19 [STEP DRIVE EN KP20]", "DO 20 [KP21 Y44.1 OPEN]", "DO 21 [ KP22 Y44.1 CLOSE]", "DO 22 [ KP23 Y44.2 OPEN]", "DO 23", "DO 24 [STEP DRIVE 1]", "DO 25 [STEP DRIVE 2]"] ("#DO")
        n100 = Multiply(x=u32 1000, y="Time, ms") -> (x*y=w166:u32)
        n101 = for {
          shift-right: [w177] -> w173
          shift-left: w171 -> [w179]
          shift-right: [w176] -> w172
          shift-left: w170 -> [w178]
          tunnel: w169 -> [w175] mode=indexing
          tunnel: w166 -> [w174]
          n102 = call "Write Do.vi"("FPGA API in"=w179, "#DO"=w175, "value"=FALSE, "Time uSec"=w174, "error in (no error)"=w178) -> ("FPGA API out"=w177:refnum<class "FPGA API.lvclass">, "error out"=w176:errorcluster)  [unwired: 9 in]
        }
      }
    }
    n103 = case shown="True" w114 {
      tunnel: [w212 w223] -> w111
      tunnel: [w211 w222] -> w99
      tunnel: w71 -> [w212 w220]
      tunnel: w70 -> [w211 w217]
      tunnel: w112 -> [_ w221]
      frame False {
      }
      frame True {
        n104 = local write "Enable Stop Drive"(FALSE ("Enable Stop Drive")) -> ()
        n105 = local write "Enable Close Outlet"(FALSE ("Enable Close Outlet")) -> ()
        n106 = local write "Enable Close Inlet"(FALSE ("Enable Close Inlet")) -> ()
        n107 = call "SetHasckelAO.vi"("FPGA API in"=w220, "Haskel in"=0.0, "error in (no error)"=w217) -> ("FPGA API out"=w219:refnum<class "FPGA API.lvclass">, "error out"=w216:errorcluster)  [unwired: 11 in]
        n108 = for {
          shift-right: [w226] -> w223
          shift-left: w219 -> [w228]
          shift-right: [w225] -> w222
          shift-left: w216 -> [w227]
          tunnel: w221 -> [w224] mode=indexing
          n109 = call "Write Do.vi"("FPGA API in"=w228, "#DO"=w224, "value"=FALSE, "Time uSec"=u32 0, "error in (no error)"=w227) -> ("FPGA API out"=w226:refnum<class "FPGA API.lvclass">, "error out"=w225:errorcluster)  [unwired: 9 in]
        }
      }
    }
    n110 = local write "error out"(w99) -> ()
    n111 = node-c288() -> ()  [unwired: 1 in, 1 out]
  }
  n112 = local write "Enable Stop Drive"(FALSE ("Enable Stop Drive")) -> ()
  n113 = local write "Enable Close Outlet"(FALSE ("Enable Close Outlet")) -> ()
  n114 = local write "Enable Close Inlet"(FALSE ("Enable Close Inlet")) -> ()
  n115 = node-c288(w12) -> ()  [unwired: 1 out]
  n116 = call "Close.vi"("FPGA API in"=w15, "error in (no error)"=w14) -> ("error out"=→"error out":errorcluster)  [unwired: 12 in, 1 out]
